vi "niRFUtil MEAS Compute Measurement Bandwidth.vi"(1 "Sampling Rate (Hz)":dbl format="%^.6e", 7 "Meas Recommended BW (Hz)":dbl format="%^.6e") -> (8 "Computed Meas BW (Hz)":dbl format="%^.6e")   [LabVIEW 2015, in "niRFUtil.lvlib"]
doc: "(c) Copyright 2006, National Instruments, Inc. This VI may not be duplicated, sold, or distributed without written consent from National Instruments."
uses:
  niRFUtil.lvlib
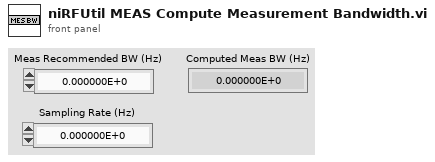
[diagram p1: front panel]
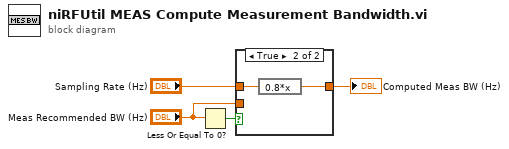
[diagram p0: block diagram]
diagram:
  n1 = Less Or Equal To 0?(x="Meas Recommended BW (Hz)") -> (x <= 0?=w4:bool)
  n2 = case shown="True" w4 {
    tunnel: "Sampling Rate (Hz)" -> [_ w7]
    tunnel: [w5 w6] -> w2
    tunnel: "Meas Recommended BW (Hz)" -> [w5 _]
    frame False {
    }
    frame True {
      n3 = expression code="0.8*x"(w7) -> (w6:dbl)
    }
  }
  "Computed Meas BW (Hz)" <- w2
